vi "CSDB_Transfer.write DB.vi"(4 "error in (no error)":errorcluster, 5 "Data array":string[][](array[string]), 6 "Instances & Classes":string[][](array[string]), 7 "Data source":string) -> (0 "error out":errorcluster)   [LabVIEW 2014, in "CSDB_Transfer.lvlib"]
doc: "Writes the Data shown on the frontpanel to the Database.\nClasses are created if necessary but without Attributes (only BaseProcess Attributes until now). If an instance already exists, the user has the option to overwrite it. (In this case all data of the instance is deleted before the new data is written.)"
uses:
  CSDB_Transfer.lvlib
  <vilib>/addons/database/Connection.llb/DB Tools Open Connec (String).vi
  <vilib>/addons/database/Connection.llb/Conn Execute.vi
  <vilib>/addons/database/Recordset.llb/Rec Destroy - Connection.vi
  <vilib>/addons/database/NI_Database_API.lvlib
  CSDB_Common/CSDB_Common.lvlib
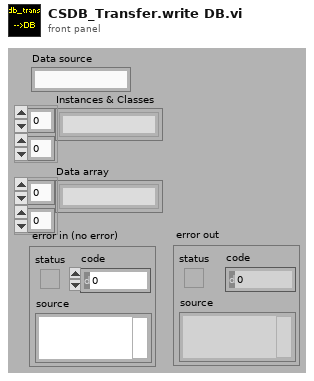
[diagram p1: front panel]
types:
  T1 = typedef "NI_Database_API.lvlib/Conn ObjectReference.ctl" = refnum<k1>
  T2 = typedef "NI_Database_API.lvlib/Rec ObjectReference.ctl" = refnum<k1>
  T3 = cluster{i32, "first element":string, "first element":string, string, string}
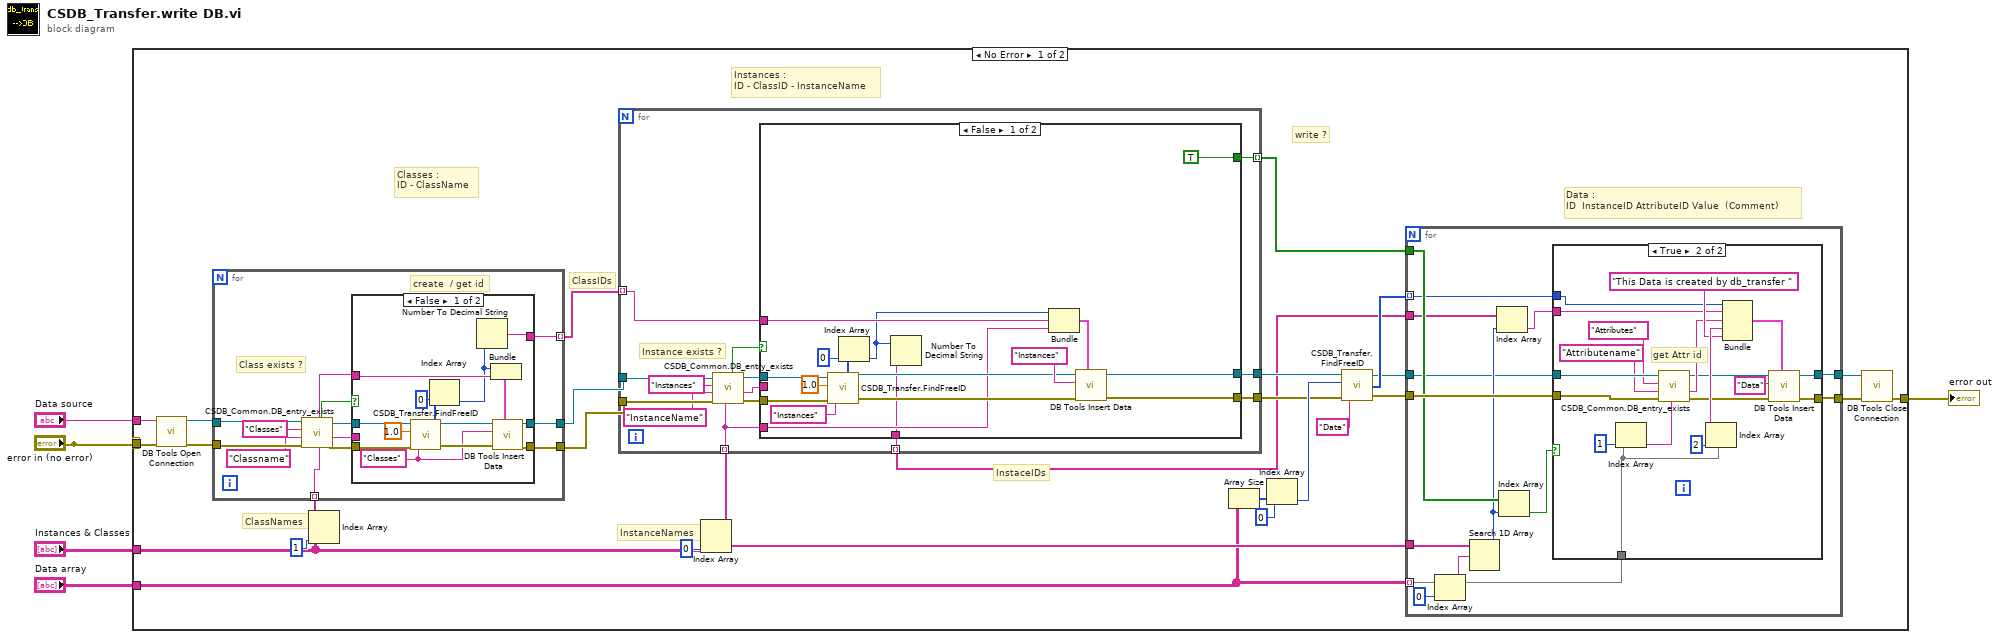
[diagram p0: block diagram]
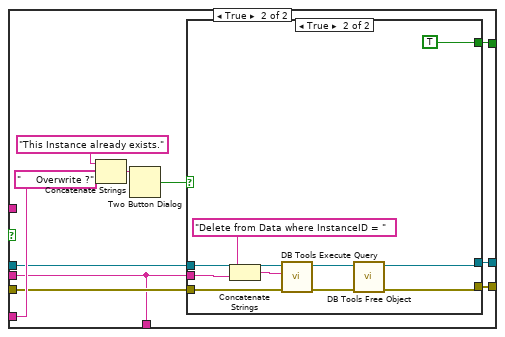
[diagram p3: hidden frame]
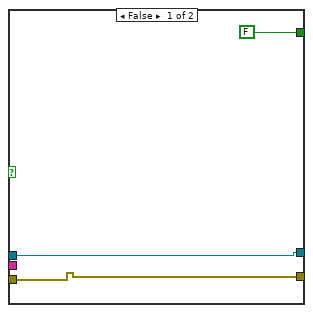
[diagram p4: hidden frame]
diagram:
  n1 = case shown="No Error" "error in (no error)" {
    selector: "error in (no error)" -> [_ w152]
    tunnel: [w24 w152] -> w5
    tunnel: "Instances & Classes" -> [w9 _]
    tunnel: "Data source" -> [w8 _]
    tunnel: "Data array" -> [w7 _]
    tunnel: "error in (no error)" -> [w6 _]
    frame No Error {
      # "InstaceIDs"
      # "write ?"
      # "Instances :\nID - ClassID - InstanceName"
      # "Classes : \nID - ClassName"
      # "InstanceNames"
      # "ClassIDs"
      # "ClassNames"
      # "Data :\nID  InstanceID AttributeID Value  (Comment)"
      n2 = call-poly <vilib>:"DB Tools Open Connection.vi"("error in (no error)"=w6, "connection information"=w8) -> ("error out"=w31:errorcluster, "connection reference"=w32:T1)  [unwired: 6 in]
      n3 = Index Array(array=w9, index (col)=1 ("disabled index (col)")) -> (element=w29:string[])  [unwired: 1 in]
      n4 = for {
        tunnel: w32 -> [w134]
        tunnel: w31 -> [w133]
        tunnel: [w127] -> w28
        tunnel: [w126] -> w27
        tunnel: w29 -> [w125] mode=indexing
        tunnel: [w124] -> w25 mode=indexing
        # "create  / get id"
        # "Class exists ?"
        n5 = call "CSDB_Common.DB_entry_exists.vi"("= (value)"=w125, "error in (no error)"=w133, "where (coloumn)"="Classname", "from (Table)"="Classes", "connection reference"=w134) -> ("error out"=w128:errorcluster, "first element"=w123:string, "connection reference out"=w129:T1, "exists ?"=w130:bool)  [unwired: 1 in, 1 out]
        n6 = case shown="False" w130 {
          tunnel: w129 -> [w148 w151]
          tunnel: w128 -> [w147 w150]
          tunnel: w125 -> [w141 _]
          tunnel: [w138 w151] -> w127
          tunnel: [w137 w150] -> w126
          tunnel: [w136 w149] -> w124
          tunnel: w123 -> [_ w149]
          frame False {
            w139 = "Classes" ("table")
            n7 = call "CSDB_Transfer.FindFreeID.vi"("error in (no error)"=w147, "table"=w139, "# of IDs"=1.0, "connection reference"=w148) -> ("error out"=w142:errorcluster, "FreeIDs"=w145:i32[], "connection reference out"=w143:T1)
            n8 = Index Array(array=w145, index=0) -> (element=w135:i32)
            n9 = Number To Decimal String(number=w135) -> (decimal integer string=w136:string)  [unwired: 1 in]
            n10 = Bundle(w135, w141) -> (w140:cluster{i32, string})  [unwired: 1 in]
            n11 = call <vilib>:"DB Tools Insert Data.vi"("data"=w140, "error in (no error)"=w142, "table"=w139, "connection reference"=w143) -> ("error out"=w137:errorcluster, "connection reference out"=w138:T1)  [unwired: 6 in]
          }
          frame True {
          }
        }
      }
      n12 = Index Array(array=w9, index (col)=0 ("disabled index (col)")) -> (element=w21:string[])  [unwired: 1 in]
      n13 = for {
        tunnel: w28 -> [w81]
        tunnel: w27 -> [w80]
        tunnel: w21 -> [w73] mode=indexing
        tunnel: w25 -> [w74] mode=indexing
        tunnel: [w72] -> w20 mode=indexing
        tunnel: [w71] -> w15
        tunnel: [w70] -> w13
        tunnel: [w68] -> w10 mode=indexing
        # "Instance exists ?"
        n14 = call "CSDB_Common.DB_entry_exists.vi"("= (value)"=w73, "error in (no error)"=w80, "where (coloumn)"="InstanceName", "from (Table)"="Instances", "connection reference"=w81) -> ("error out"=w75:errorcluster, "first element"=w69:string, "connection reference out"=w76:T1, "exists ?"=w77:bool)  [unwired: 1 in, 1 out]
        n15 = case shown="False" w77 {
          tunnel: w76 -> [w92 w102]
          tunnel: w75 -> [w91 w100]
          tunnel: w74 -> [w88 _]
          tunnel: w73 -> [w87 w107]
          tunnel: [TRUE w104] -> w72
          tunnel: [w85 w103] -> w71
          tunnel: [w84 w101] -> w70
          tunnel: w69 -> [_ w99]
          tunnel: [w82 w99] -> w68
          frame False {
            n16 = call "CSDB_Transfer.FindFreeID.vi"("error in (no error)"=w91, "table"="Instances", "# of IDs"=1.0, "connection reference"=w92) -> ("error out"=w89:errorcluster, "FreeIDs"=w95:i32[], "connection reference out"=w90:T1)
            n17 = Index Array(array=w95, index=0) -> (element=w83:i32)
            n18 = Number To Decimal String(number=w83) -> (decimal integer string=w82:string)  [unwired: 1 in]
            n19 = Bundle(w83, "first element"=w88, w87) -> (w93:cluster{i32, "first element":string, string})  [unwired: 1 in]
            n20 = call <vilib>:"DB Tools Insert Data.vi"("data"=w93, "error in (no error)"=w89, "table"="Instances", "connection reference"=w90) -> ("error out"=w84:errorcluster, "connection reference out"=w85:T1)  [unwired: 6 in]
          }
          frame True {
            n21 = Concatenate Strings("This Instance already exists.", w107, "     Overwrite ?" ("string")) -> (w109:string)
            n22 = Two Button Dialog(message=w109) -> (T button?=w105:bool)  [unwired: 2 in]
            n23 = case shown="True" w105 {
              tunnel: [FALSE TRUE] -> w104
              tunnel: [w111 w116] -> w103
              tunnel: w102 -> [w111 w119]
              tunnel: [w110 w117] -> w101
              tunnel: w100 -> [w110 w118]
              tunnel: w99 -> [_ w114]
              frame False {
              }
              frame True {
                n24 = Concatenate Strings("Delete from Data where InstanceID = ", w114) -> (w115:string)
                n25 = call-poly <vilib>:"DB Tools Execute Query.vi"("error in (no error)"=w118, "SQL query"=w115, "connection reference"=w119) -> ("error out"=w120:errorcluster, "recordset reference"=w121:T2)  [unwired: 5 in]
                n26 = call-poly <vilib>:"DB Tools Free Object.vi"("error in (no error)"=w120, "recordset reference"=w121) -> ("error out"=w117:errorcluster, "connection reference"=w116:T1)  [unwired: 8 in]
              }
            }
          }
        }
      }
      n27 = Array Size(array=w7) -> (size(s)=w19:i32[])
      n28 = Index Array(array=w19, index=0) -> (element=w16:i32)
      n29 = call "CSDB_Transfer.FindFreeID.vi"("error in (no error)"=w13, "table"="Data", "# of IDs"=w16, "connection reference"=w15) -> ("error out"=w14:errorcluster, "FreeIDs"=w12:i32[], "connection reference out"=w11:T1)
      n30 = for {
        tunnel: w7 -> [w41] mode=indexing
        tunnel: w14 -> [w46]
        tunnel: [w45] -> w22
        tunnel: [w44] -> w23
        tunnel: w21 -> [w43]
        tunnel: w20 -> [w38]
        tunnel: w10 -> [w37]
        tunnel: w11 -> [w34]
        tunnel: w12 -> [w33] mode=indexing
        n31 = Index Array(array=w41, index=0) -> (element=w40:string)
        n32 = Search 1D Array(1D array=w43, element=w40) -> (index of element=w36:i32)  [unwired: 1 in]
        n33 = Index Array(array=w37, index=w36) -> (element=w35:string)
        n34 = Index Array(array=w38, index=w36) -> (element=w39:bool)
        n35 = case shown="True" w39 {
          tunnel: w34 -> [w48 w58]
          tunnel: w46 -> [w47 w57]
          tunnel: [w48 w62] -> w45
          tunnel: [w47 w61] -> w44
          tunnel: w41 -> [_ w59]
          tunnel: w35 -> [_ w52]
          tunnel: w33 -> [_ w49]
          frame False {
          }
          frame True {
            # "get Attr id"
            n36 = Index Array(array=w59, index=1) -> (element=w54:string)
            n37 = call "CSDB_Common.DB_entry_exists.vi"("= (value)"=w54, "error in (no error)"=w57, "where (coloumn)"="Attributename", "from (Table)"="Attributes", "connection reference"=w58) -> ("error out"=w50:errorcluster, "first element"=w53:string, "connection reference out"=w51:T1)  [unwired: 1 in, 2 out]
            n38 = Index Array(array=w59, index=2) -> (element=w65:string)
            n39 = Bundle(w49, "first element"=w52, "first element"=w53, w65, "This Data is created by db_transfer ") -> (w64:T3)  [unwired: 1 in]
            n40 = call <vilib>:"DB Tools Insert Data.vi"("data"=w64, "error in (no error)"=w50, "table"="Data", "connection reference"=w51) -> ("error out"=w61:errorcluster, "connection reference out"=w62:T1)  [unwired: 6 in]
          }
        }
      }
      n41 = call <vilib>:"DB Tools Close Connection.vi"("error in (no error)"=w23, "connection reference"=w22) -> ("error out"=w24:errorcluster)  [unwired: 5 in]
    }
    frame Error {
    }
  }
  "error out" <- w5
